vi "Void.vi"(8 "Error In":errorcluster) -> (0 "Error Out":errorcluster)   [LabVIEW 2017, in "Tests.lvlib" / "From Msgpack.lvlib"]
uses:
  From Msgpack.lvlib
  <vilib>/addons/_JKI Toolkits/Caraya/classes/Test/Test.lvclass
  src/LabPack/LabPack.lvlib
  <vilib>/addons/_JKI Toolkits/Caraya/classes/Assert/Assert.lvclass
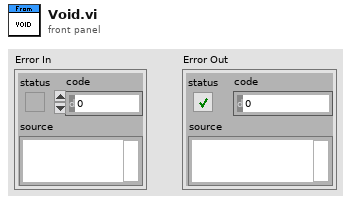
[diagram p1: front panel]
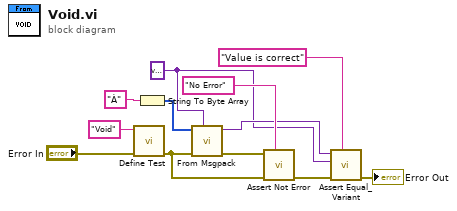
[diagram p0: block diagram]
diagram:
  w1 = variant
  n1 = call <vilib>:"Define Test.vi"("error in (no error)"="Error In", "Label (VI Title)"="Void") -> ("error out"=w8:errorcluster)  [unwired: 9 in]
  n2 = String To Byte Array(string="À") -> (unsigned byte array=w10:u8[])
  n3 = call "From Msgpack.vi"("Types and Defaults"=w1, "Error In"=w8, "Msgpack Data"=w10) -> ("Error Out"=w9:errorcluster, "Value"=w2:variant)  [unwired: 7 in]
  n4 = call <vilib>:"Assert Not Error.vi"("Label"="No Error", "error in (no error)"=w8, "Not Error?"=w9) -> ("error out"=w7:errorcluster)  [unwired: 8 in]
  n5 = call <vilib>:"Assert Equal_Variant.vi"("Label"="Value is correct", "error in (no error)"=w7, "Y"=w1, "X"=w2) -> ("error out"=→"Error Out":errorcluster)  [unwired: 7 in]
